vi "电机控制__SR830_LOCKIN_V0.1.9.vi"() -> ()   [LabVIEW 2015]
uses:
  <vilib>/Utility/file.llb/Write To Spreadsheet File (DBL).vi
panel:
  in  "选项卡控件":enum32{"Motor", "SCAN_Spectrum"}(tab)
  in  "ComPort":i16=2
  in  "axis":i16
  in  "AxisStyle":i16
  in  "AccSpeed":sgl=1000.0
  in  "InitSpeed":sgl=1000.0
  in  "dir":i16
  in  "workstate":i16=1
  in  "Speed":sgl=1000.0
  in  "step":sgl=1000.0
  in  "StepAngle":sgl
  in  "x":sgl=2000.0
  in  "state":i16=1
  out "字符串":string="打开失败"
  in  "Motor Port":i8=2 min=0
  in  "sampling interval":u32=100 min=1 max=500000
  in  "Sampling number":i32=1000
  out "Lock_in String Received":string
  out "时域波形图":cluster{"Y":dbl[], "Y":dbl[]}[](graph)
  out "字符串 2":string="打开失败"
  in  "dir 2":i16=1
  in  "AxisStyle 2":i16
  in  "AccSpeed 2":sgl
  in  "Speed 2":sgl=1000.0
  in  "InitSpeed 2":sgl=1000.0
  in  "step 2":sgl=1000.0
  in  "StepAngle 2":sgl
  in  "workstate 2":i16=1
  in  "state 2":i16=1
  in  "baud rate (9600)":u32=9600 caption="波特率"
  in  "VISA resource name":refnum<visa-resource-name> caption="LOCKIN VISA"
  in  "stop bits (10: 1 bit)":u16(ring)=10 caption="停止位（10: 1位）" items=["1.0"=10, "1.5"=15, "2.0"=20]
  in  "data bits (8)":u16=8 caption="数据比特(8)" min=5 max=8 step=1
  in  "parity (0:none)":enum16{"None", "Odd", "Even", "Mark", "Space"}(ring) caption="奇偶（0:无）"
  out "LOCKIN OK":bool
  in  "Motor  Axis":u8
  in  "Scan times":i32
  in  "file path (dialog if empty) 2":path caption="多次扫描数据文件路径 （空时为对话框）"
  in  "motor step len":dbl=2.5
  out "out1*1000":dbl
  out "读取缓冲区2":string
  out "字符串 3":string="打开失败"
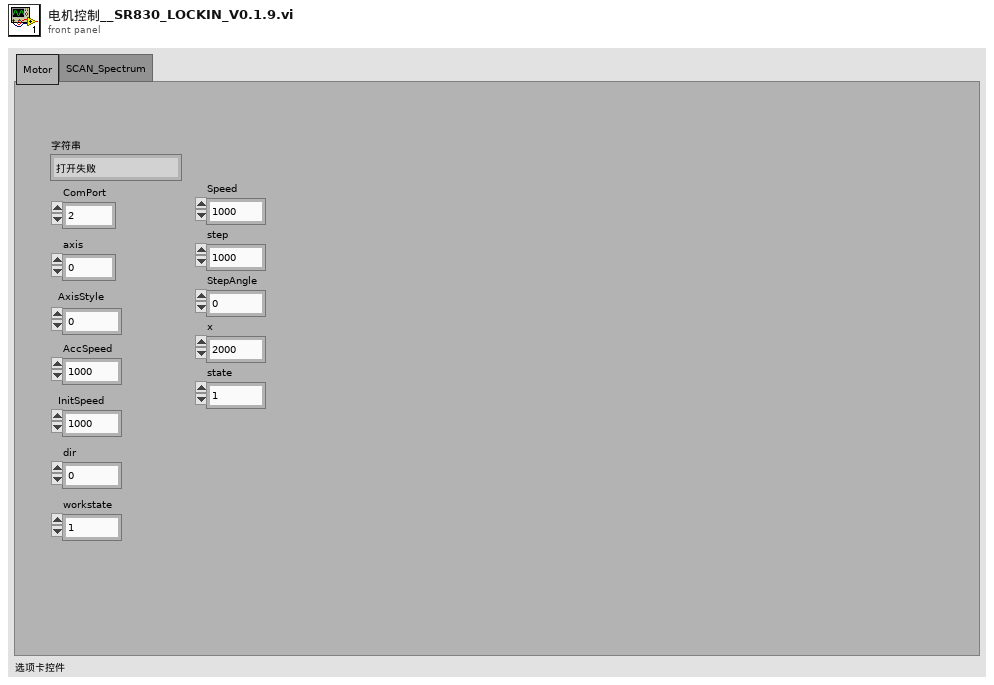
[diagram p1: front panel]
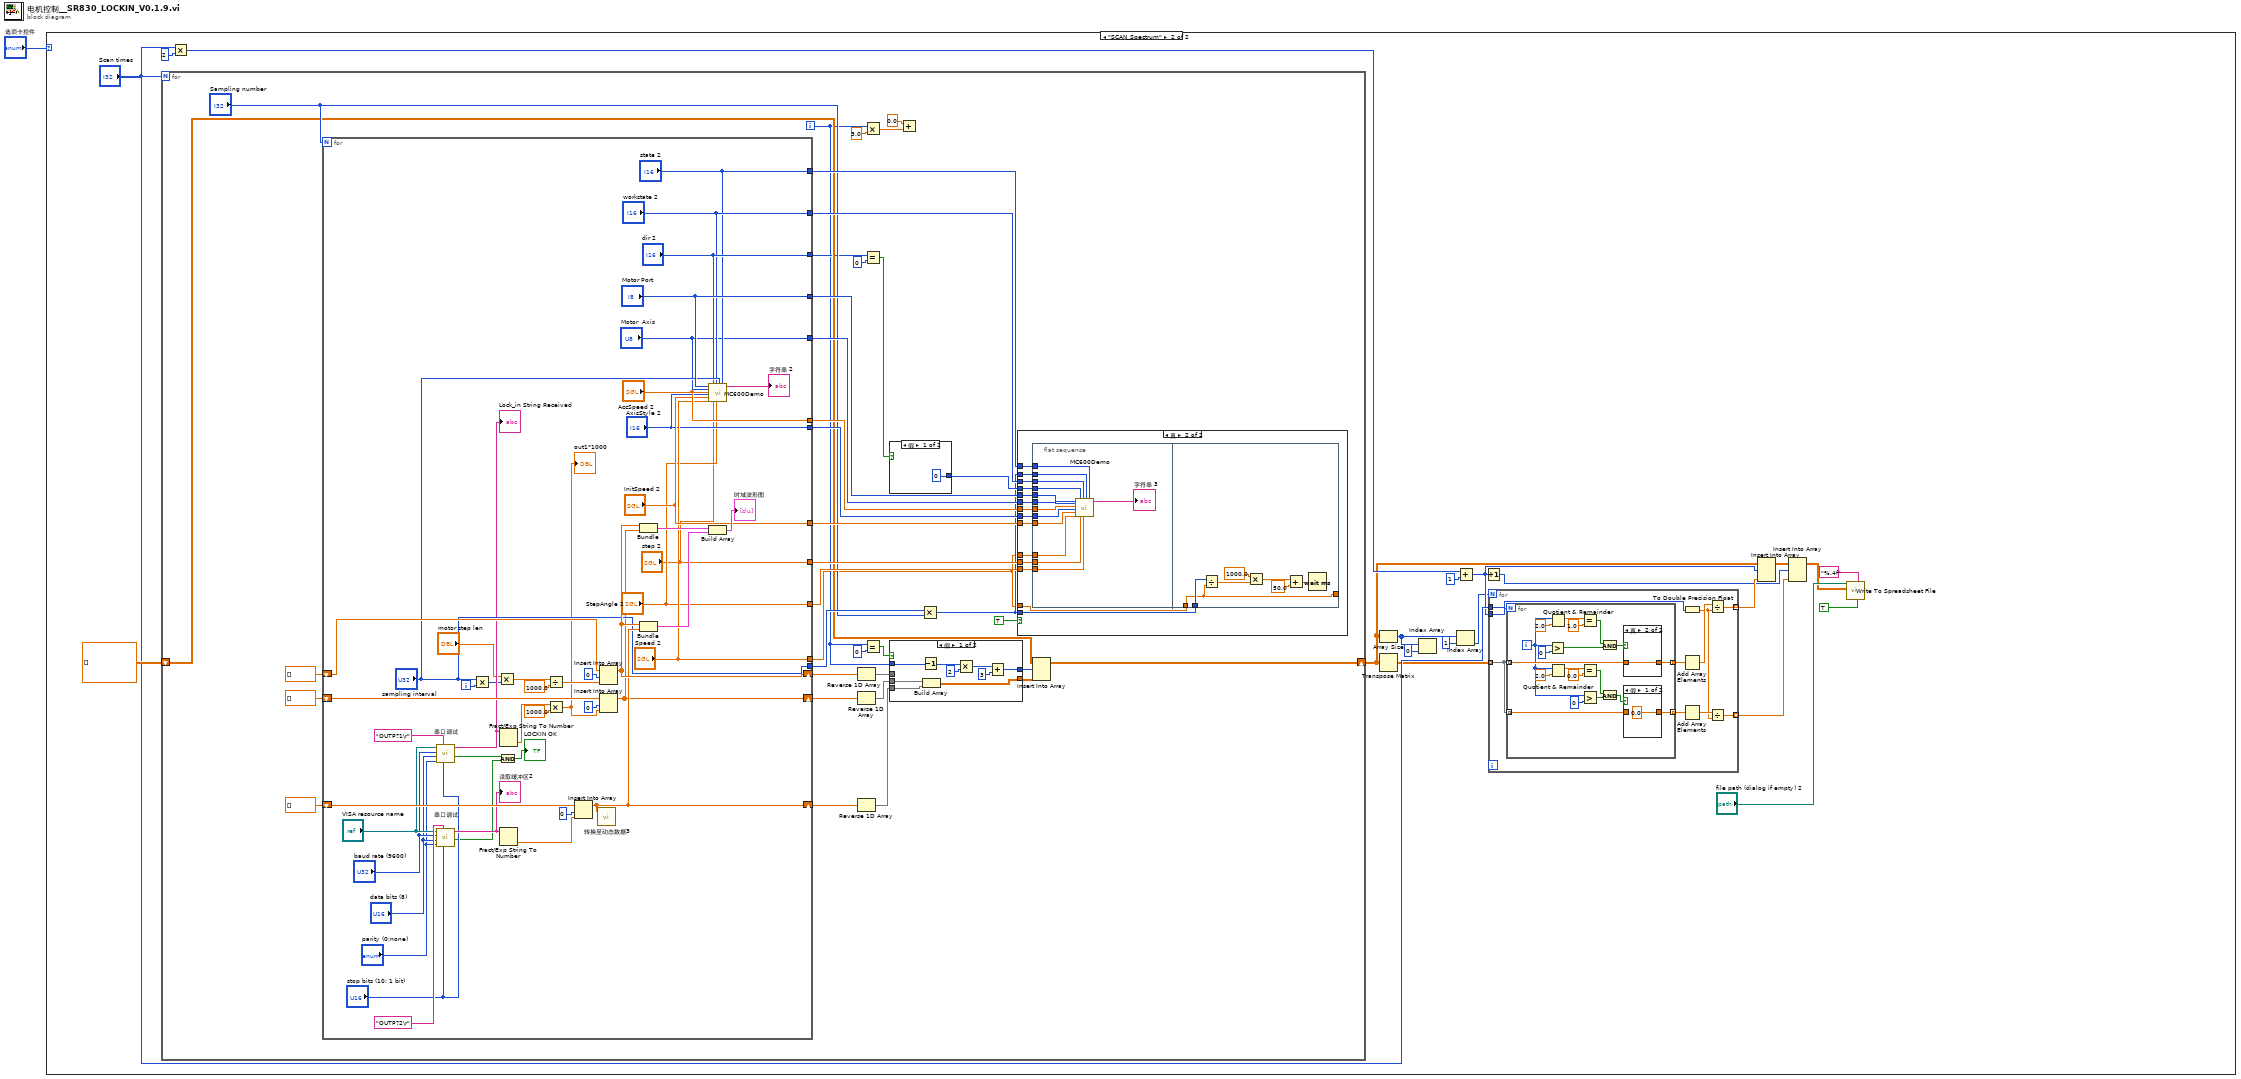
[diagram p0: block diagram]
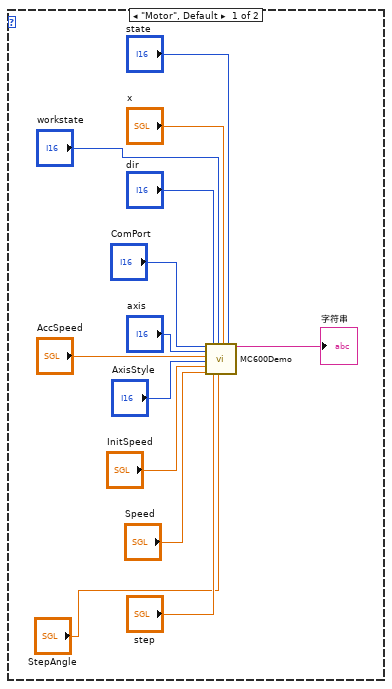
[diagram p2: hidden frame]
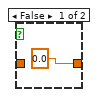
[diagram p4: hidden frame]
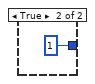
[diagram p5: hidden frame]
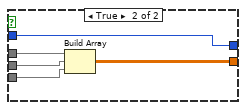
[diagram p6: hidden frame]
diagram:
  n1 = case shown="\"SCAN_Spectrum\"" "选项卡控件" {
    frame "Motor", Default {
      n2 = call "MC600Demo.vi"("ComPort"="ComPort", "axis"="axis", "AccSpeed"="AccSpeed", "AxisStyle"="AxisStyle", "InitSpeed"="InitSpeed", "Speed"="Speed", "dir"="dir", "step"="step", "workstate"="workstate", "StepAngle"="StepAngle", "x"="x", "state"="state") -> ("字符串"=→"字符串":string)  [unwired: 7 in]
    }
    frame "SCAN_Spectrum" {
      n3 = for {
        N: "Scan times" -> [_]
        shift-right: [w85] -> w18
        shift-left: dbl[][] [] -> [w86]
        i -> [w74]
        n4 = for {
          N: "Sampling number" -> [_]
          tunnel: ["Motor Port"] -> w103
          tunnel: ["Motor  Axis"] -> w102
          tunnel: ["sampling interval"] -> w88
          shift-right: [w194] -> w99
          shift-left: dbl[] [] -> [w201]
          shift-right: [w157] -> w98
          shift-left: dbl[] [] -> [w200]
          shift-right: [w193] -> w96
          shift-left: dbl[] [] -> [w196]
          tunnel: ["dir 2"] -> w78
          tunnel: ["AccSpeed 2"] -> w95
          tunnel: ["InitSpeed 2"] -> w94
          tunnel: ["Speed 2"] -> w68
          tunnel: ["AxisStyle 2"] -> w93
          tunnel: ["StepAngle 2"] -> w92
          tunnel: ["workstate 2"] -> w91
          tunnel: ["state 2"] -> w90
          tunnel: ["step 2"] -> w89
          i -> [w198]
          n5 = call "串口调试.vi"("stop bits (10: 1 bit)"="stop bits (10: 1 bit)", "写入缓冲区"="OUTP?1\r" ("Command String"), "parity (0:none)"="parity (0:none)", "data bits (8)"="data bits (8)", "baud rate (9600)"="baud rate (9600)", "VISA resource name"="VISA resource name") -> ("OK"=w155:bool, "读取缓冲区"=w177:string)  [unwired: 4 in]
          "Lock_in String Received" <- w177
          n6 = call "串口调试.vi"("stop bits (10: 1 bit)"="stop bits (10: 1 bit)", "写入缓冲区"="OUTP?2\r" ("Command String"), "parity (0:none)"="parity (0:none)", "data bits (8)"="data bits (8)", "baud rate (9600)"="baud rate (9600)", "VISA resource name"="VISA resource name") -> ("OK"=w168:bool, "读取缓冲区"=w175:string)  [unwired: 4 in]
          "读取缓冲区2" <- w175
          n7 = Multiply(x="sampling interval", y=w198) -> (x*y=w162:u32)
          n8 = Multiply(x="motor step len", y=w162) -> (x*y=w164:dbl)
          n9 = And(x=w155, y=w168) -> (x .and. y?=→"LOCKIN OK":bool)
          n10 = Fract/Exp String To Number(string=w177) -> (number=w160:dbl)  [unwired: 3 in, 1 out]
          n11 = Fract/Exp String To Number(string=w175) -> (number=w156:dbl)  [unwired: 3 in, 1 out]
          n12 = Divide(x=w164, y=1000.0) -> (x/y=w165:dbl)
          n13 = Multiply(x=w160, y=1000.0) -> (x*y=w158:dbl)
          "out1*1000" <- w158
          n14 = Insert Into Array(array=w196, index=0 ("索引"), new element=w156) -> (w193:dbl[])
          n15 = call "转换至动态数据3"("Array"=w193) -> ()  [unwired: 3 in, 1 out]
          n16 = Insert Into Array(array=w201, index=0 ("索引"), new element=w165) -> (w194:dbl[])
          n17 = Insert Into Array(array=w200, index=0 ("索引"), new element=w158) -> (w157:dbl[])
          n18 = Bundle(w194, w157) -> (w192:cluster{dbl[], dbl[]})  [unwired: 1 in]
          n19 = Bundle(w194, w193) -> (w191:cluster{dbl[], dbl[]})  [unwired: 1 in]
          n20 = call "MC600Demo.vi"("ComPort"="Motor Port", "axis"="Motor  Axis", "AccSpeed"="AccSpeed 2", "AxisStyle"="AxisStyle 2", "InitSpeed"="InitSpeed 2", "Speed"="Speed 2", "dir"="dir 2", "step"="step 2", "workstate"="workstate 2", "StepAngle"="StepAngle 2", "x"="sampling interval", "state"="state 2") -> ("字符串"=→"字符串 2":string)  [unwired: 7 in]
          n21 = Build Array(w192, w191) -> (→"时域波形图":cluster{dbl[], dbl[]}[])
        }
        n22 = Reverse 1D Array(array=w99) -> (reversed array=w82:dbl[])
        n23 = Reverse 1D Array(array=w98) -> (reversed array=w81:dbl[])
        n24 = Reverse 1D Array(array=w96) -> (reversed array=w80:dbl[])
        n25 = Multiply(x=w74, y=3.0) -> (x*y=w72:dbl)
        n26 = Equal?(x=w78, y=i16 0) -> (x = y?=w79:bool)
        n27 = Equal?(x=w74, y=0) -> (x = y?=w84:bool)
        n28 = case shown="假" w79 {
          tunnel: [i16 0 ("y") i16 1 ("y")] -> w76
          frame False {
          }
          frame True {
          }
        }
        n29 = case shown="假" w84 {
          tunnel: w82 -> [_ w120]
          tunnel: w81 -> [w107 w119]
          tunnel: w80 -> [w108 w118]
          tunnel: [w115 w117] -> w70
          tunnel: w74 -> [w110 w116]
          tunnel: [w111 w116] -> w71
          frame False {
            n30 = Decrement(x=w110) -> (x-1=w109:i32)
            n31 = Build Array(w107, w108) -> (w115:dbl[][])
            n32 = Multiply(x=w109, y=2) -> (x*y=w113:i32)
            n33 = Add(x=w113, y=3) -> (x+y=w111:i32)
          }
          frame True {
            n34 = Build Array(w120, w119, w118) -> (w117:dbl[][])
          }
        }
        n35 = Add(x=0.0, y=w72) -> ()  [unwired: 1 out]
        n36 = Multiply(x=w88, y="Sampling number") -> (x*y=w69:u32)
        n37 = case shown="真" TRUE ("back to start") {
          tunnel: w103 -> [_ w123]
          tunnel: w102 -> [_ w124]
          tunnel: w76 -> [_ w131]
          tunnel: w69 -> [_ w133]
          tunnel: w95 -> [_ w125]
          tunnel: w94 -> [_ w127]
          tunnel: w68 -> [_ w128]
          tunnel: w93 -> [_ w126]
          tunnel: w92 -> [_ w130]
          tunnel: w91 -> [_ w132]
          tunnel: w90 -> [_ w134]
          tunnel: w89 -> [_ w129]
          tunnel: w69 -> [_ w122]
          tunnel: w68 -> [_ w121]
          frame False {
          }
          frame True {
            n38 = flat-sequence {
              tunnel: w134 -> [w147]
              tunnel: w133 -> [w146]
              tunnel: w132 -> [w145]
              tunnel: w131 -> [w144]
              tunnel: w130 -> [w143]
              tunnel: w129 -> [w142]
              tunnel: w128 -> [w141]
              tunnel: w127 -> [w140]
              tunnel: w126 -> [w139]
              tunnel: w125 -> [w138]
              tunnel: w124 -> [w137]
              tunnel: w123 -> [w136]
              tunnel: w122 -> [w154]
              tunnel: [w153] -> _
              tunnel: w121 -> [w153]
              frame #0 {
                n39 = call "MC600Demo.vi"("ComPort"=w136, "axis"=w137, "AccSpeed"=w138, "AxisStyle"=w139, "InitSpeed"=w140, "Speed"=w141, "dir"=w144, "step"=w142, "workstate"=w145, "StepAngle"=w143, "x"=w146, "state"=w147) -> ("字符串"=→"字符串 3":string)  [unwired: 7 in]
              }
              frame #1 {
                n40 = Divide(x=w154, y=w153) -> (x/y=w152:sgl)
                n41 = Multiply(x=sgl 1000.0, y=w152) -> (x*y=w149:sgl)
                n42 = Add(x=w149, y=sgl 50.0) -> (x+y=w151:sgl)
                n43 = Wait (ms)(milliseconds to wait=w151) -> ()  [unwired: 1 out]
              }
            }
          }
        }
        n44 = Insert Into Array(array=w86, index (row)=w71, new element=w70) -> (w85:dbl[][])  [unwired: 1 in]
      }
      n45 = Multiply(x="Scan times", y=2) -> (x*y=w21:i32)
      n46 = Array Size(array=w18) -> (size(s)=w32:i32[])
      n47 = Transpose Matrix(1:w18) -> (0:w17:dbl[][])
      n48 = Index Array(array=w32, index=0 ("索引")) -> ()  [unwired: 1 out]
      n49 = Index Array(array=w32, index=1 ("索引")) -> (element=w16:i32)
      n50 = Add(x=w21, y=1) -> (x+y=w19:i32)
      n51 = Increment(x=w19) -> (x+1=w25:i32)
      n52 = for {
        N: w16 -> [_]
        tunnel: w17 -> [w40] mode=indexing
        tunnel: "Scan times" -> [w36]
        tunnel: w19 -> [w44]
        tunnel: [w41] -> w26 mode=indexing
        tunnel: [w37] -> w24 mode=indexing
        n53 = for {
          N: w44 -> [_]
          tunnel: [w55] -> w43 mode=indexing
          tunnel: w40 -> [w56] mode=indexing
          tunnel: w40 -> [w46] mode=indexing
          tunnel: [w45] -> w39 mode=indexing
          i -> [w48]
          n54 = Greater?(x=w48, y=0) -> (0:w62:bool)
          n55 = Quotient & Remainder(x=w48, y=2.0) -> (x-y*floor(x/y)=w58:dbl)  [unwired: 1 out]
          n56 = Quotient & Remainder(x=w48, y=2.0) -> (x-y*floor(x/y)=w53:dbl)  [unwired: 1 out]
          n57 = Equal?(x=w58, y=1.0) -> (x = y?=w60:bool)
          n58 = Equal?(x=w53, y=0.0) -> (x = y?=w51:bool)
          n59 = Greater?(x=w48, y=0) -> (0:w50:bool)
          n60 = And(x=w60, y=w62) -> (x .and. y?=w61:bool)
          n61 = And(x=w51, y=w50) -> (x .and. y?=w47:bool)
          n62 = case shown="真" w61 {
            tunnel: w56 -> [_ w67]
            tunnel: [0.0 w67] -> w55
            frame False {
            }
            frame True {
            }
          }
          n63 = case shown="假" w47 {
            tunnel: w46 -> [_ w65]
            tunnel: [0.0 w65] -> w45
            frame False {
            }
            frame True {
            }
          }
        }
        n64 = Add Array Elements(numeric array=w43) -> (sum=w42:dbl)
        n65 = Add Array Elements(numeric array=w39) -> (sum=w38:dbl)
        n66 = To Double Precision Float(number=w36) -> (double precision float=w35:dbl)
        n67 = Divide(x=w42, y=w35) -> (x/y=w41:dbl)
        n68 = Divide(x=w38, y=w35) -> (x/y=w37:dbl)
      }
      n69 = Insert Into Array(array=w18, index (row)=w19, new element=w26) -> (w27:dbl[][])  [unwired: 1 in]
      n70 = Insert Into Array(array=w27, index (row)=w25, new element=w24) -> (w15:dbl[][])  [unwired: 1 in]
      n71 = call-poly <vilib>:"Write To Spreadsheet File.vi"("transpose? (no:F)"=TRUE, "format (%.3f)"="%.4f", "2D data"=w15, "file path (dialog if empty)"="file path (dialog if empty) 2") -> ()  [unwired: 4 in, 1 out]
    }
  }
